vi "Write Result Data.vi"(8 "error in (no error)":errorcluster, 10 "Result Data":refnum<class "HGF_VariantDataObject.lvclass">, 11 "HGF_DataAnalysis in":refnum<class "HGF_DataAnalysis.lvclass">) -> (0 "error out":errorcluster, 3 "HGF_DataAnalysis out":refnum<class "HGF_DataAnalysis.lvclass">)   [LabVIEW 2012, in "HGF_DataAnalyzer.lvlib" / "HGF_DataAnalysis.lvclass"]
uses:
  HGF_DataAnalysis.lvclass
  HGF_LVC/HGF_BaseClasses/HGF_VariantDataObject/HGF_VariantDataObject.lvclass
  HGF_DataAnalysis.lvclass/HGF_DataAnalysis.ctl
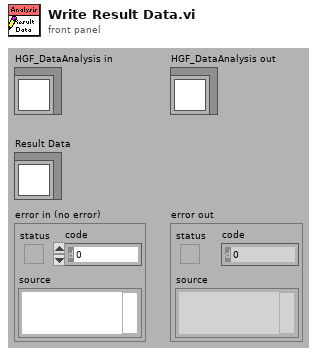
[diagram p1: front panel]
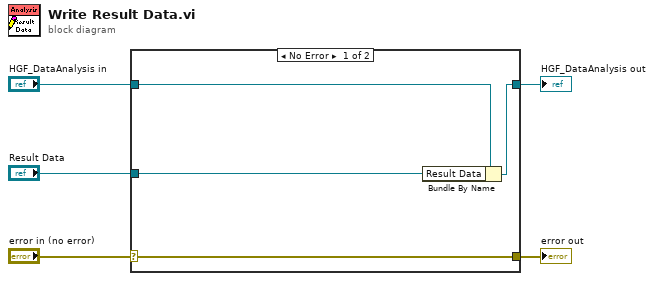
[diagram p0: block diagram]
diagram:
  n1 = case shown="No Error" "error in (no error)" {
    selector: "error in (no error)" -> [w9 w10]
    tunnel: [w9 w10] -> w4
    tunnel: [w7 w11] -> w2
    tunnel: "HGF_DataAnalysis in" -> [w8 w11]
    tunnel: "Result Data" -> [w6 _]
    frame No Error {
      n2 = Bundle By Name(cluster=w8, "Result Data"=w6) -> (w7:refnum<class "HGF_DataAnalysis.lvclass">)
    }
    frame Error {
    }
  }
  "error out" <- w4
  "HGF_DataAnalysis out" <- w2
